vi "Import data --subVI.vi"(8 "error in (no error)":errorcluster, 11 "String":string) -> (0 "error out":errorcluster, 3 "Array":cluster{"Angle":dbl, "Data":dbl}[](array[cluster]))   [LabVIEW 2020]
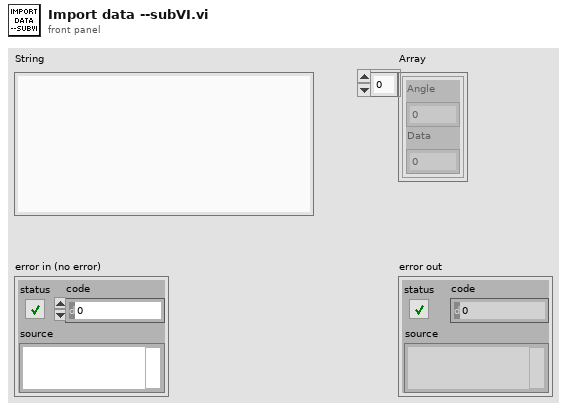
[diagram p1: front panel]
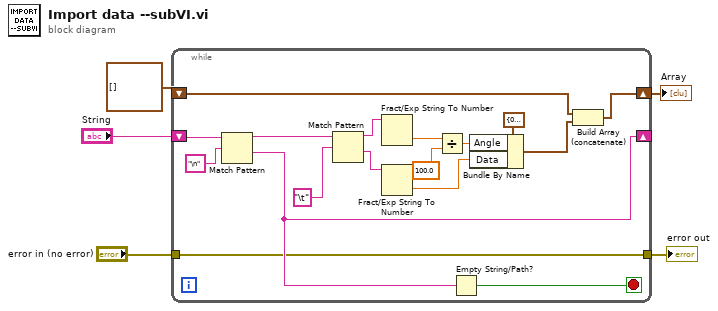
[diagram p0: block diagram]
diagram:
  n1 = while {
    shift-right: [w12] -> w3
    shift-left: cluster{"Angle":dbl, "Data":dbl}[] [] -> [w11]
    shift-right: [w10] -> _
    shift-left: "String" -> [w19]
    tunnel: [w9] -> w1
    tunnel: "error in (no error)" -> [w9]
    stop <- w18 stop-if-true
    n2 = Match Pattern(string=w19, regular expression="\n") -> (before substring=w21:string, after substring=w10:string)  [unwired: 1 in, 2 out]
    n3 = Match Pattern(string=w21, regular expression="\t") -> (before substring=w17:string, after substring=w16:string)  [unwired: 1 in, 2 out]
    n4 = Fract/Exp String To Number(string=w17) -> (number=w8:dbl)  [unwired: 3 in, 1 out]
    n5 = Fract/Exp String To Number(string=w16) -> (number=w14:dbl)  [unwired: 3 in, 1 out]
    n6 = Divide(x=w8, y=100.0) -> (x/y=w7:dbl)
    n7 = Empty String/Path?(string/path=w10) -> (empty?=w18:bool)
    n8 = Bundle By Name(cluster=cluster{"Angle":dbl, "Data":dbl} {"Angle"=0.0, "Data"=0.0} ("Angle vs V"), "Angle"=w7, "Data"=w14) -> (w13:cluster{"Angle":dbl, "Data":dbl})
    n9 = Build Array (concatenate)(w11, w13) -> (w12:cluster{"Angle":dbl, "Data":dbl}[])
  }
  "Array" <- w3
  "error out" <- w1
